vi "Get Type.vi"(8 "error in (no error)":errorcluster, 11 "Chemicals in":refnum<class "Chemicals.lvclass">) -> (0 "error out":errorcluster, 2 "Item Type":T1, 3 "Chemicals out":refnum<class "Chemicals.lvclass">)   [LabVIEW 2020, in "Chemicals.lvclass"]
uses:
  Chemicals.lvclass
  Item/Item Type.ctl
  Item/Item.lvclass
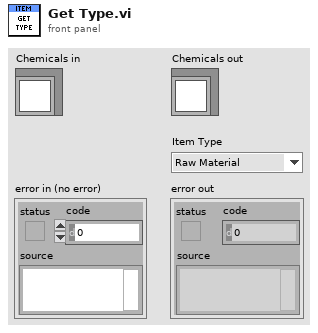
[diagram p1: front panel]
types:
  T1 = typedef "Item.lvclass/Item Type.ctl" = enum16{"Raw Material", "Component", "Module", "Product"}
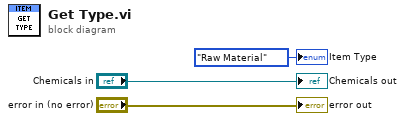
[diagram p0: block diagram]
diagram:
  "error out" <- "error in (no error)"
  "Chemicals out" <- "Chemicals in"
  "Item Type" <- Item_Type."Raw Material" ("Item Type")
